vi "ws_users Template Keys.vi"(6 "Current User Record":T1, 7 "Edit sxUsername (\"\")":string, 8 "error in (no error)":errorcluster, 9 "Copy? (f)":bool, 10 "Edit? (f)":bool, 11 "Connection Refnum":T2) -> (0 "error out":errorcluster, 1 "Template Keys":T3, 3 "Connection Refnum":T2)   [LabVIEW 2011]
uses:
  <vilib>/addons/internet/utils/keyedarr.llb/Keyed Array.ctl
  SI.LIB/ODBC/SQL Controls/Connection Refnum.ctl
  server/database/Users/User Record.ctl
  <vilib>/addons/internet/utils/strutil.llb/Case Matching.ctl
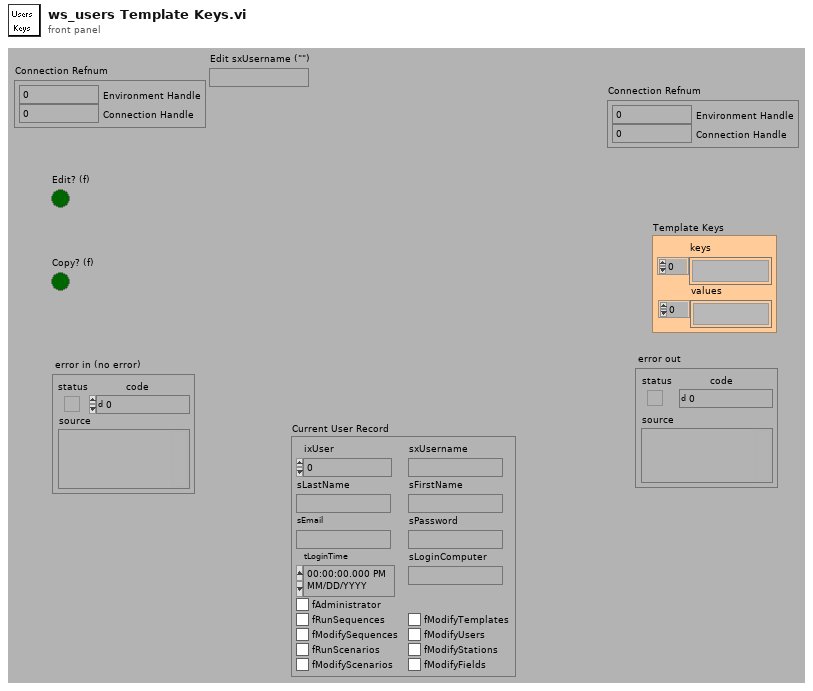
[diagram p1: front panel]
types:
  T1 = typedef "User Record.ctl" = cluster{"ixUser":i32, "sxUsername":string, "sLastName":string, "sFirstName":string, "sEmail":string, "sPassword":string, "tLoginTime":timestamp, "sLoginComputer":string, "fAdministrator":bool, "fRunSequences":bool, "fModifySequences":bool, "fRunScenarios":bool, "fModifyScenarios":bool, "fModifyTemplates":bool, "fModifyUsers":bool, "fModifyStations":bool, "fModifyFields":bool}
  T2 = typedef "Connection Refnum.ctl" = cluster{"Environment Handle":i32, "Connection Handle":i32}
  T3 = typedef "Keyed Array.ctl" = cluster{"keys":string[], "values":string[]}
  T4 = typedef "Case Matching.ctl" = enum16{"a != A", "a == A", "system"}
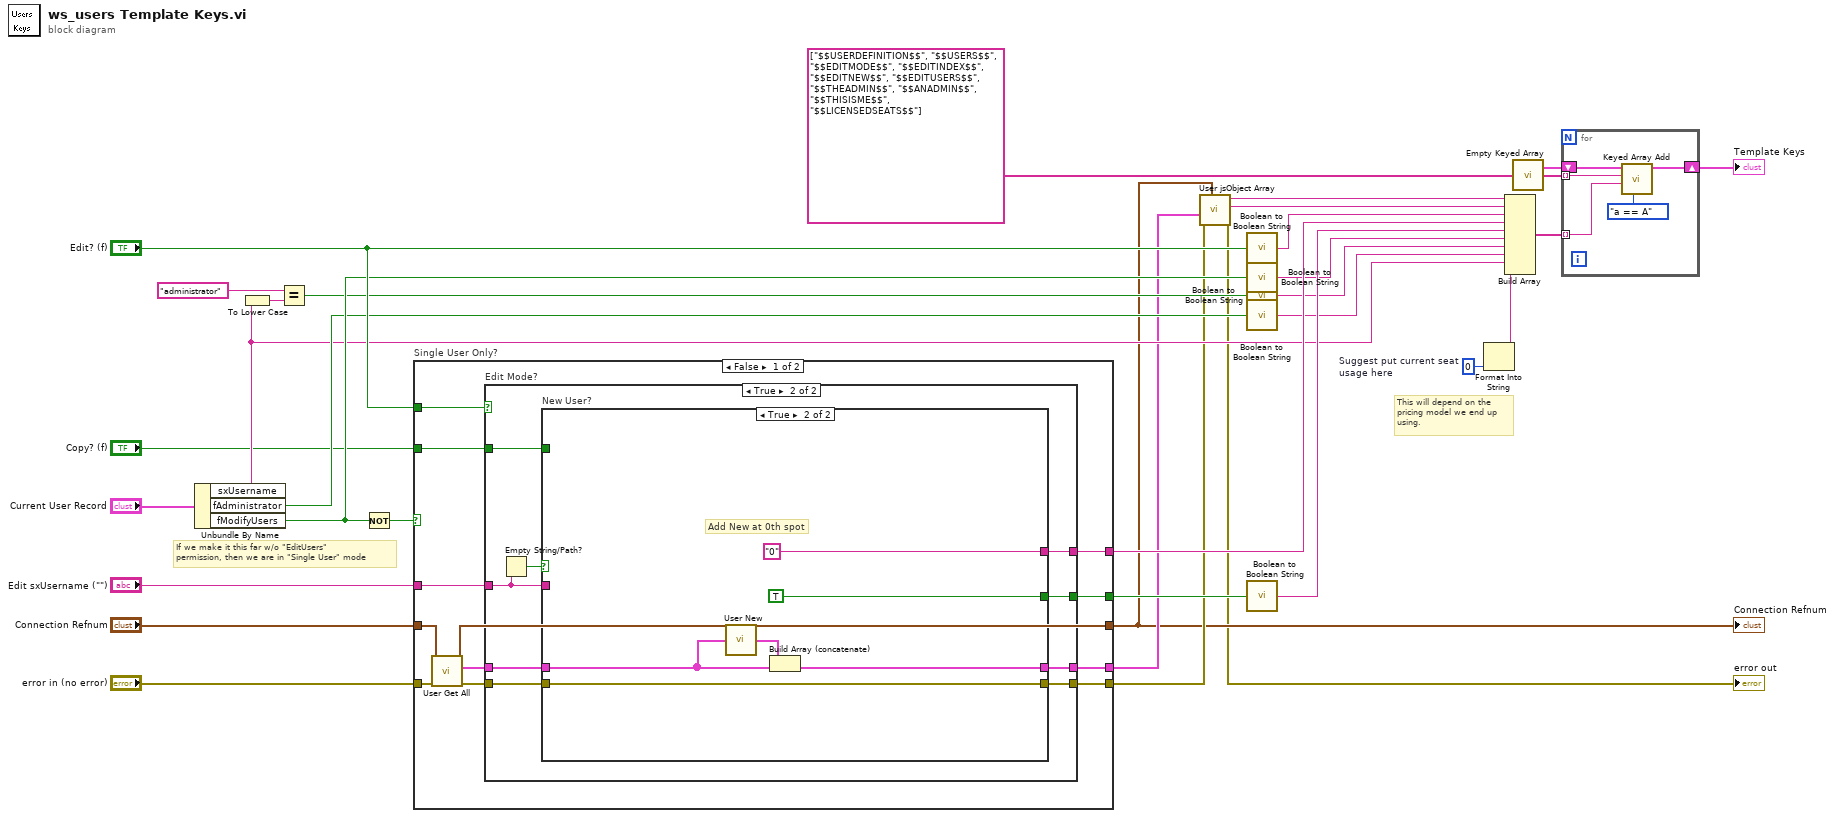
[diagram p0: block diagram]
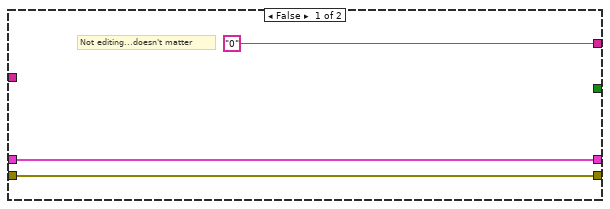
[diagram p2: hidden frame]
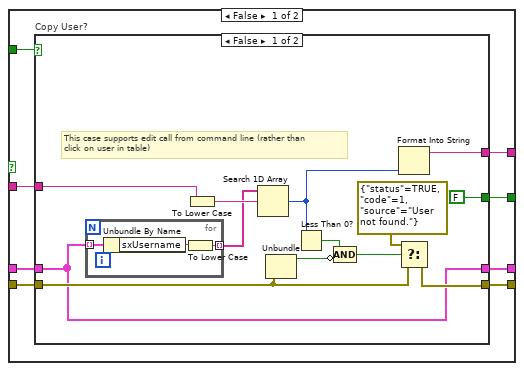
[diagram p3: hidden frame]
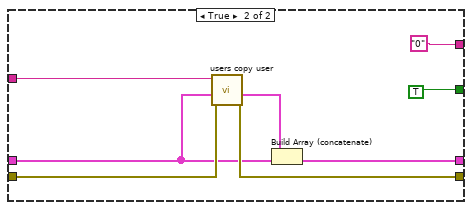
[diagram p4: hidden frame]
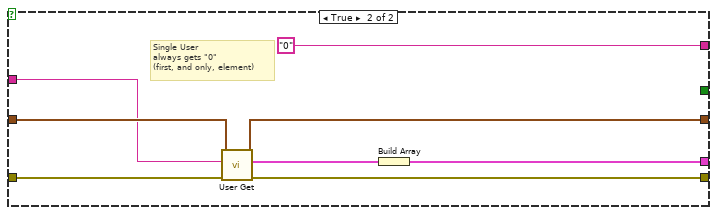
[diagram p5: hidden frame]
diagram:
  w1 = 0  # Suggest put current seat usage here
  # "This will depend on the\npricing model we end up\nusing."
  # "If we make it this far w/o \"EditUsers\"\npermission, then we are in \"Single User\" mode"
  n1 = Unbundle By Name("Current User Record") -> ("sxUsername"=w10:string, "fAdministrator"=w16:bool, "fModifyUsers"=w18:bool)
  n2 = To Lower Case(string=w10) -> (all lower case string=w14:string)
  n3 = Equal?(x="administrator", y=w14) -> (x = y?=w11:bool)
  n4 = Not(x=w18) -> (.not. x?=w24:bool)
  n5 = case "Single User Only?" shown="False" w24 {
    tunnel: "Connection Refnum" -> [w44 w98]
    tunnel: "error in (no error)" -> [w43 w101]
    tunnel: [w39 w102] -> w6
    tunnel: [w37 w100] -> w7
    tunnel: [w42 w97] -> w3
    tunnel: "Edit sxUsername (\"\")" -> [w35 w96]
    tunnel: [w36 "0"] -> w22
    tunnel: "Edit? (f)" -> [w40 _]
    tunnel: [w34 _] -> w19
    tunnel: "Copy? (f)" -> [w33 _]
    frame False {
      n6 = call "User Get All.vi"("error in (no error)"=w43, "Connection Refnum"=w44) -> ("error out"=w38:errorcluster, "User Records"=w41:T1[], "Connection Refnum"=w42:T2)  [unwired: 2 in, 5 out]
      n7 = case "Edit Mode?" shown="True" w40 {
        tunnel: w41 -> [w47 w56]
        tunnel: [w47 w52] -> w39
        tunnel: w38 -> [w46 w54]
        tunnel: [w46 w53] -> w37
        tunnel: ["0" w51] -> w36
        tunnel: w35 -> [_ w50]
        tunnel: [_ w49] -> w34
        tunnel: w33 -> [_ w48]
        frame False {
          # "Not editing...doesn't matter"
        }
        frame True {
          n8 = Empty String/Path?(string/path=w50) -> (empty?=w55:bool)
          n9 = case "New User?" shown="True" w55 {
            tunnel: w56 -> [w63 w89]
            tunnel: w54 -> [w60 w94]
            tunnel: [w61 w94] -> w53
            tunnel: [w57 w92] -> w52
            tunnel: [w62 "0"] -> w51
            tunnel: w50 -> [w64 _]
            tunnel: [w58 TRUE] -> w49
            tunnel: w48 -> [w59 _]
            frame False {
              n10 = case "Copy User?" shown="False" w59 {
                tunnel: w64 -> [w75 w82]
                tunnel: w63 -> [w65 w81]
                tunnel: [w73 "0"] -> w62
                tunnel: [w72 w85] -> w61
                tunnel: w60 -> [w71 w86]
                tunnel: [FALSE TRUE] -> w58
                tunnel: [w65 w83] -> w57
                frame False {
                  # "This case supports edit call from command line (rather than\nclick on user in table)"
                  n11 = for {
                    tunnel: w65 -> [w80] mode=indexing
                    tunnel: [w78] -> w76 mode=indexing
                    n12 = Unbundle By Name(w80) -> ("sxUsername"=w79:string)
                    n13 = To Lower Case(string=w79) -> (all lower case string=w78:string)
                  }
                  n14 = To Lower Case(string=w75) -> (all lower case string=w77:string)
                  n15 = Search 1D Array(1D array=w76, element=w77) -> (index of element=w74:i32)  [unwired: 1 out]
                  n16 = Unbundle(w71) -> ("status"=w70:bool)  [unwired: 2 out]
                  n17 = Less Than 0?(x=w74) -> (x < 0?=w69:bool)
                  n18 = Compound Arithmetic op=AND(w69, invert w70) -> (w68:bool)
                  n19 = Format Into String(w74) -> (resulting string=w73:string)  [unwired: 3 in, 1 out]
                  n20 = Select(t=errorcluster {"status"=TRUE, "code"=1, "source"="User not found."}, s=w68, f=w71) -> (s? t:f=w72:errorcluster)
                }
                frame True {
                  n21 = call "users copy user.vi"("error in (no error)"=w86, "All Users (empty)"=w81, "sxUsername (\"\")"=w82) -> ("error out"=w85:errorcluster, "User Information"=w84:T1)  [unwired: 7 out]
                  n22 = Build Array (concatenate)(w84, w81) -> (w83:T1[])
                }
              }
            }
            frame True {
              # "Add New at 0th spot"
              n23 = call "User New.vi"("Existing User Records (empty)"=w89) -> ("Default New User"=w93:T1)
              n24 = Build Array (concatenate)(w93, w89) -> (w92:T1[])
            }
          }
        }
      }
    }
    frame True {
      # "Single User \nalways gets \"0\"\n(first, and only, element)"
      n25 = call "User Get.vi"("error in (no error)"=w101, "sxUsername (\"\")"=w96, "Connection Refnum"=w98) -> ("error out"=w100:errorcluster, "User"=w99:T1, "Connection Refnum"=w97:T2)  [unwired: 6 out]
      n26 = Build Array(w99) -> (w102:T1[])
    }
  }
  "Connection Refnum" <- w3
  n27 = call "User jsObject Array.vi"("DB Connection Ref"=w3, "error in (no error)"=w7, "USERS (empty)"=w6) -> ("error out"=→"error out":errorcluster, "Users jsObject Array"=w5:string, "User jsObject Definition"=w4:string)  [unwired: 3 in, 3 out]
  n28 = call "Boolean to Boolean String.vi"("Boolean"="Edit? (f)") -> ("Boolean string"=w26:string)  [unwired: 1 in]
  n29 = call "Boolean to Boolean String.vi"("Boolean"=w18) -> ("Boolean string"=w17:string)  [unwired: 1 in]
  n30 = call "Boolean to Boolean String.vi"("Boolean"=w11) -> ("Boolean string"=w12:string)  [unwired: 1 in]
  n31 = call "Boolean to Boolean String.vi"("Boolean"=w16) -> ("Boolean string"=w15:string)  [unwired: 1 in]
  n32 = call "Boolean to Boolean String.vi"("Boolean"=w19) -> ("Boolean string"=w20:string)  [unwired: 1 in]
  n33 = Format Into String(w1) -> (resulting string=w9:string)  [unwired: 3 in, 1 out]
  n34 = Build Array(w4, w5, w26, w22, w20, w17, w12, w15, w10, w9) -> (w29:string[])
  n35 = call "Empty Keyed Array.vi"() -> ("empty keyed array"=w32:T3)  [unwired: 3 out]
  n36 = for {
    shift-right: [w104] -> w30
    shift-left: w32 -> [w106]
    tunnel: string[] ["$$USERDEFINITION$$", "$$USERS$$", "$$EDITMODE$$", "$$EDITINDEX$$", "$$EDITNEW$$", "$$EDITUSERS$$", "$$THEADMIN$$", "$$ANADMIN$$", "$$THISISME$$", "$$LICENSEDSEATS$$"] -> [w105] mode=indexing
    tunnel: w29 -> [w103] mode=indexing
    n37 = call <vilib>:"Keyed Array Add.vi"("case matching (sensitive)"=Case_Matching."a == A", "value"=w103, "key"=w105, "array in"=w106) -> ("array out"=w104:T3)  [unwired: 3 out]
  }
  "Template Keys" <- w30
